vi "Read Parameters.vi"(8 "error in (no error)":errorcluster, 11 "PID in":refnum<class "PID.lvclass">) -> (0 "error out":errorcluster, 2 "Parameters":T1, 3 "PID out":refnum<class "PID.lvclass">)   [LabVIEW 2020, in "IG PID.lvlib" / "PID.lvclass"]
uses:
  PID.lvclass
  Parameters.ctl
  PID.lvclass/PID.ctl
  IG PID.lvlib
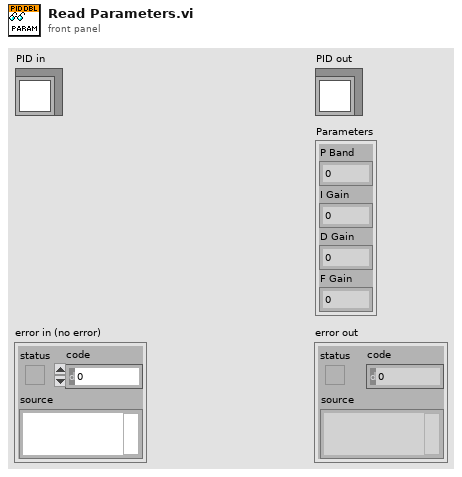
[diagram p1: front panel]
types:
  T1 = typedef "IG PID.lvlib/Parameters.ctl" = cluster{"P Band":dbl, "I Gain":dbl, "D Gain":dbl, "F Gain":dbl}
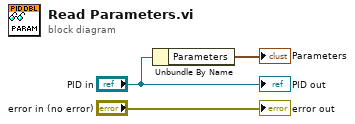
[diagram p0: block diagram]
diagram:
  n1 = Unbundle By Name("PID in") -> ("Parameters"=→"Parameters":T1)
  "error out" <- "error in (no error)"
  "PID out" <- "PID in"
